vi "Create Channel Lookup.vi"(8 "error in (no error)":errorcluster, 11 "VolatusAPI in":refnum<class "VolatusAPI.lvclass">) -> (0 "error out":errorcluster, 3 "VolatusAPI out":refnum<class "VolatusAPI.lvclass">)   [LabVIEW 2020, in "Volatus.lvlib" / "VolatusAPI.lvclass"]
uses:
  VolatusAPI.lvclass
  lv-vecto/Vecto/Channel Info.ctl
  VolatusAPI.lvclass/VolatusAPI.ctl
  VolatusConfig/VolatusConfigElement/VolatusConfigElement.lvclass/VolatusConfigElement.ctl
  VolatusConfig/VolatusConfigElement/Element.vi
  VolatusConfig/VolatusConfigElement/Lookup Child by Name.vi
  VolatusConfig/Node/Node Config.lvclass
  C:/dev/lv20CE/relink/lv-volatus/VolatusConfig/VolatusConfigElement/VolatusConfigElement.lvclass
  VolatusConfig/Task/Task Config.lvclass
  VolatusConfig/Group/Group Config.lvclass
  VolatusConfig/Channel/Channel Config.lvclass
  lv-cdm/CDM-Config/Config Element/Lookup Child by Name.vi
  lv-cdm/CDM-Config/Config Element/Value (String).vi
  VolatusConfig/Cluster/Cluster Config.lvclass
  VolatusConfig/VolatusConfigElement/VolatusConfigElement.lvclass
  lv-vecto/VectoConfig/VectoConfig.lvlib
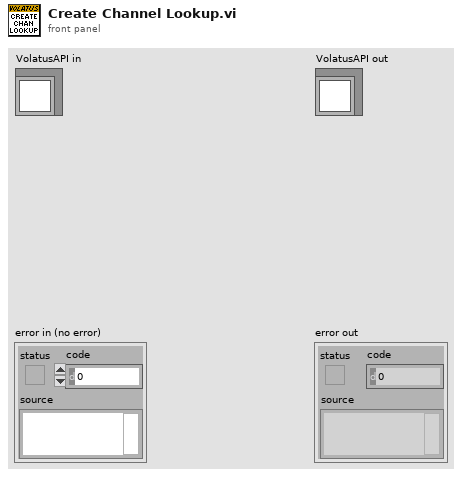
[diagram p1: front panel]
types:
  T1 = typedef "VectoConfig.lvlib/Channel Info.ctl" = cluster{"Name":string, "Group":string, "Owning Node":string, "Owning Task":string, "Resource":string}
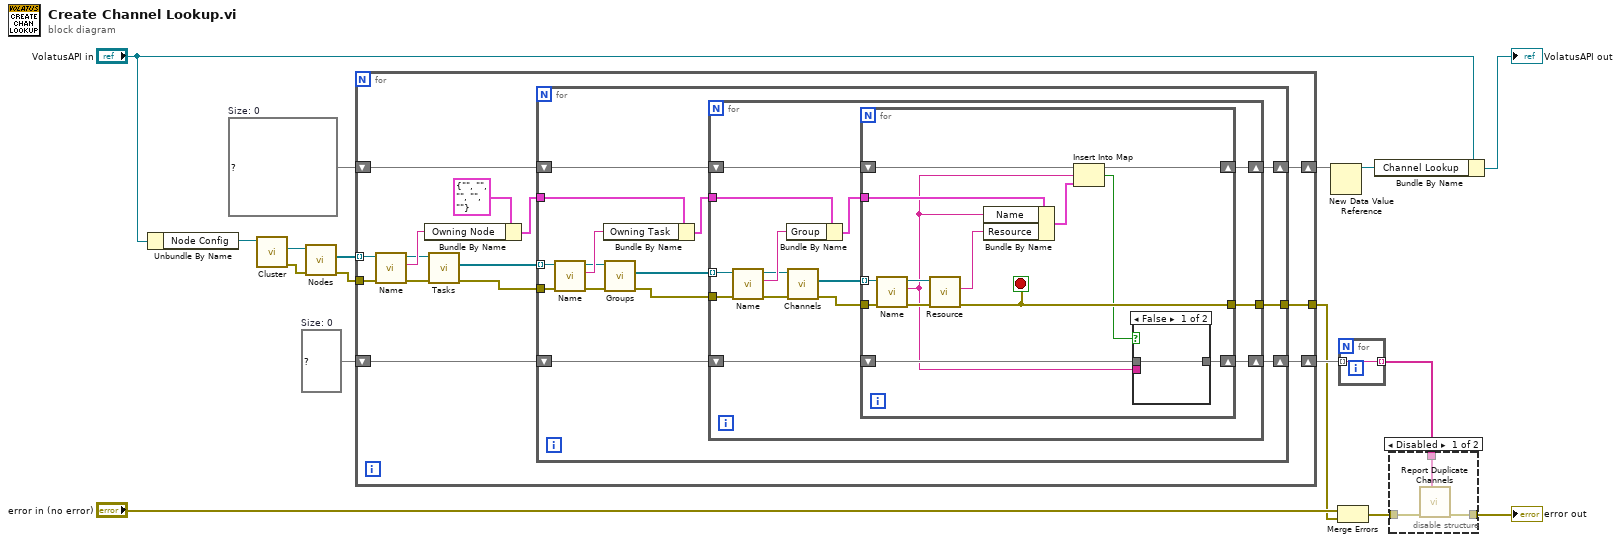
[diagram p0: block diagram]
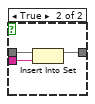
[diagram p3: hidden frame]
diagram:
  w9 = set{string} {}  # Size: 0
  w10 = map{string, T1} {}  # Size: 0
  n1 = Unbundle By Name("VolatusAPI in") -> ("Node Config"=w15:refnum<class "Node Config.lvclass">)
  n2 = call "Cluster.vi"("Node in"=w15) -> ("error out"=w13:errorcluster, "Cluster"=w14:refnum<class "Cluster Config.lvclass">)  [unwired: 8 in, 1 out]
  n3 = call "Nodes.vi"("error in (no error)"=w13, "Cluster in"=w14) -> ("error out"=w11:errorcluster, "Nodes"=w12:refnum<class "Node Config.lvclass">[])  [unwired: 7 in, 1 out]
  n4 = for {
    tunnel: w12 -> [w31] mode=indexing
    tunnel: w11 -> [w30]
    shift-right: [w21] -> w8
    shift-left: w10 -> [w22]
    shift-right: [w19] -> w5
    shift-left: w9 -> [w20]
    tunnel: [w18] -> w3
    n5 = call "Name.vi"("error in (no error)"=w30, "VolatusConfigElement in"=w31) -> ("error out"=w26:errorcluster, "Name"=w28:string, "VolatusConfigElement out"=w27:refnum<class "Node Config.lvclass">)  [unwired: 7 in]
    n6 = Bundle By Name(cluster=T1 {"Name"="", "Group"="", "Owning Node"="", "Owning Task"="", "Resource"=""} ("Channel Info"), "Owning Node"=w28) -> (w25:T1)
    n7 = call "Tasks.vi"("error in (no error)"=w26, "Node in"=w27) -> ("error out"=w23:errorcluster, "Tasks"=w24:refnum<class "Task Config.lvclass">[])  [unwired: 7 in, 1 out]
    n8 = for {
      tunnel: w25 -> [w43]
      tunnel: w24 -> [w45] mode=indexing
      tunnel: w23 -> [w44]
      shift-right: [w35] -> w21
      shift-left: w22 -> [w36]
      shift-right: [w33] -> w19
      shift-left: w20 -> [w34]
      tunnel: [w32] -> w18
      n9 = call "Name.vi"("error in (no error)"=w44, "VolatusConfigElement in"=w45) -> ("error out"=w40:errorcluster, "Name"=w42:string, "VolatusConfigElement out"=w41:refnum<class "Task Config.lvclass">)  [unwired: 7 in]
      n10 = Bundle By Name(cluster=w43, "Owning Task"=w42) -> (w37:T1)
      n11 = call "Groups.vi"("error in (no error)"=w40, "Task in"=w41) -> ("error out"=w38:errorcluster, "Groups"=w39:refnum<class "Group Config.lvclass">[])  [unwired: 7 in, 1 out]
      n12 = for {
        tunnel: w39 -> [w59] mode=indexing
        tunnel: w38 -> [w58]
        tunnel: w37 -> [w57]
        shift-right: [w49] -> w35
        shift-left: w36 -> [w50]
        shift-right: [w47] -> w33
        shift-left: w34 -> [w48]
        tunnel: [w46] -> w32
        n13 = call "Name.vi"("error in (no error)"=w58, "VolatusConfigElement in"=w59) -> ("error out"=w54:errorcluster, "Name"=w56:string, "VolatusConfigElement out"=w55:refnum<class "Group Config.lvclass">)  [unwired: 7 in]
        n14 = Bundle By Name(cluster=w57, "Group"=w56) -> (w53:T1)
        n15 = call "Channels.vi"("error in (no error)"=w54, "Group in"=w55) -> ("error out"=w51:errorcluster, "Channels"=w52:refnum<class "Channel Config.lvclass">[])  [unwired: 7 in, 1 out]
        n16 = for {
          tunnel: w53 -> [w69]
          tunnel: w52 -> [w73] mode=indexing
          tunnel: w51 -> [w72]
          shift-right: [w65] -> w49
          shift-left: w50 -> [w67]
          shift-right: [w61] -> w47
          shift-left: w48 -> [w62]
          tunnel: [w64] -> w46
          stop <- w64 stop-if-true
          n17 = call "Name.vi"("error in (no error)"=w72, "VolatusConfigElement in"=w73) -> ("error out"=w70:errorcluster, "Name"=w60:string, "VolatusConfigElement out"=w71:refnum<class "Channel Config.lvclass">)  [unwired: 7 in]
          n18 = call "Resource.vi"("error in (no error)"=w70, "Channel in"=w71) -> ("error out"=w64:errorcluster, "Resource"=w68:string)  [unwired: 7 in, 1 out]
          n19 = Bundle By Name(cluster=w69, "Name"=w60, "Resource"=w68) -> (w66:T1)
          n20 = Insert Into Map(map in=w67, key=w60, value=w66) -> (map out=w65:map{string, T1}, key already included?=w63:bool)  [unwired: 1 out]
          n21 = case shown="False" w63 {
            tunnel: w62 -> [w74 w77]
            tunnel: [w74 w76] -> w61
            tunnel: w60 -> [_ w75]
            frame False {
            }
            frame True {
              n22 = Insert Into Set(10:w75, 11:w77) -> (3:w76:set{string})  [unwired: 1 out]
            }
          }
        }
      }
    }
  }
  n23 = New Data Value Reference(data value=w8) -> (data value reference=w6:refnum<data-value>)  [unwired: 1 in, 1 out]
  n24 = Merge Errors("error in (no error)", w3) -> (w4:errorcluster)
  n25 = for {
    tunnel: w5 -> [w78] mode=indexing
    tunnel: [w78] -> w1 mode=indexing
  }
  n26 = Bundle By Name(cluster="VolatusAPI in", "Channel Lookup"=w6) -> (→"VolatusAPI out":refnum<class "VolatusAPI.lvclass">)
  n27 = disable-structure shown="Disabled" {
    disable-tunnel: w4 -> [w81 w82]
    disable-tunnel: [w80 w82] -> w2
    disable-tunnel: w1 -> [w79 _]
    frame Disabled {
      n28 = call "Report Duplicate Channels.vi"("Duplicate Channels"=w79, "error in (no error)"=w81) -> ("error out"=w80:errorcluster)  [unwired: 9 in]
    }
    frame Enabled {
    }
  }
  "error out" <- w2
